vi "Voronoi Diagram.vi"(10 "Y":dbl[](array[numeric]), 11 "X":dbl[](array[numeric])) -> (0 "error":i32, 1 "Voronoi Edges":i32[][](array[numeric]), 2 "Voronoi Y":dbl[](array[numeric]), 3 "Voronoi X":dbl[](array[numeric]))   [LabVIEW 2017, in "NI_AAL_Geometry.lvlib"]
doc: "Computes the Voronoi diagram of specified points in a plane."
uses:
  <vilib>/Analysis/NI_AAL_Geometry.lvlib
panel:
  # "Voronoi Diagram"
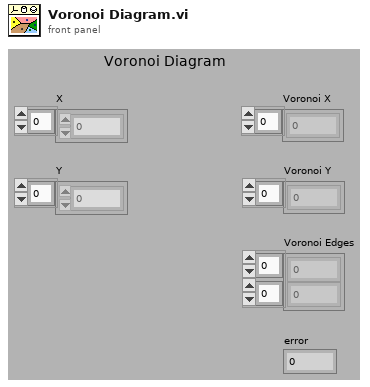
[diagram p1: front panel]
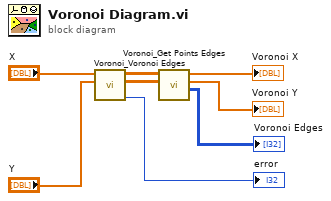
[diagram p0: block diagram]
diagram:
  n1 = call <vilib>:"Voronoi_Voronoi Edges.vi"("Y"="Y", "X"="X") -> ("error"=→"error":i32, "Edge Y"=w5:dbl[][], "Edge X"=w6:dbl[][])  [unwired: 7 in]
  n2 = call <vilib>:"Voronoi_Get Points Edges.vi"("Edge Y"=w5, "Edge X"=w6) -> ("Voronoi Edges"=→"Voronoi Edges":i32[][], "Voronoi Y"=→"Voronoi Y":dbl[], "Voronoi X"=→"Voronoi X":dbl[])  [unwired: 7 in]
